vi "_Read.vi"(8 "error in (no error)":errorcluster, 11 "Lockin and Keithley Multimeter in":refnum<class "Lockin and Keithley Multimeter.lvclass">) -> (0 "error out":errorcluster, 2 "X array":T1, 3 "Lockin and Keithley Multimeter out":refnum<class "Lockin and Keithley Multimeter.lvclass">)   [LabVIEW 2017, in "Lockin and Keithley Multimeter.lvclass"]
doc: "(Protected, Dynamic, Pure Virtual/Abstract) Perform a measurement and return one or more channels of data. Outsiders should not call this method, but instead the public \"Read Data.vi\"."
uses:
  Lockin and Keithley Multimeter.lvclass
  Utility Classes/Readable/X array.ctl
  Utility Classes/Readable/X.ctl
  Lockin and Keithley Multimeter.lvclass/Lockin and Keithley Multimeter.ctl
  Lockin/sr830/SR830.lvlib
  Utility Classes/Readable/Readable.lvclass
panel:
  out "Ratio multiplier":dbl
  out "Keithley multiplier":dbl
  out "Lockin multiplier":dbl
  out "Keithley measurement":dbl format="%^.6e"
  out "R":dbl
  out "Y":dbl
  out "X":dbl
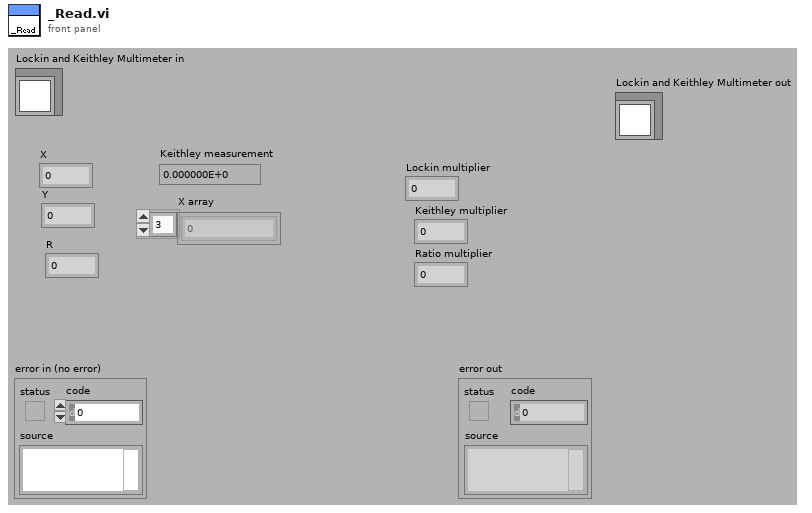
[diagram p1: front panel]
types:
  T1 = typedef "Readable.lvclass/X array.ctl" = T2[]
  T2 = typedef "Readable.lvclass/X.ctl" = dbl
  T3 = typedef "Lockin SR830.lvclass/Sensitivity.ctl" = u16
  T4 = cluster{"error":bool, "code":i32, "source":string}
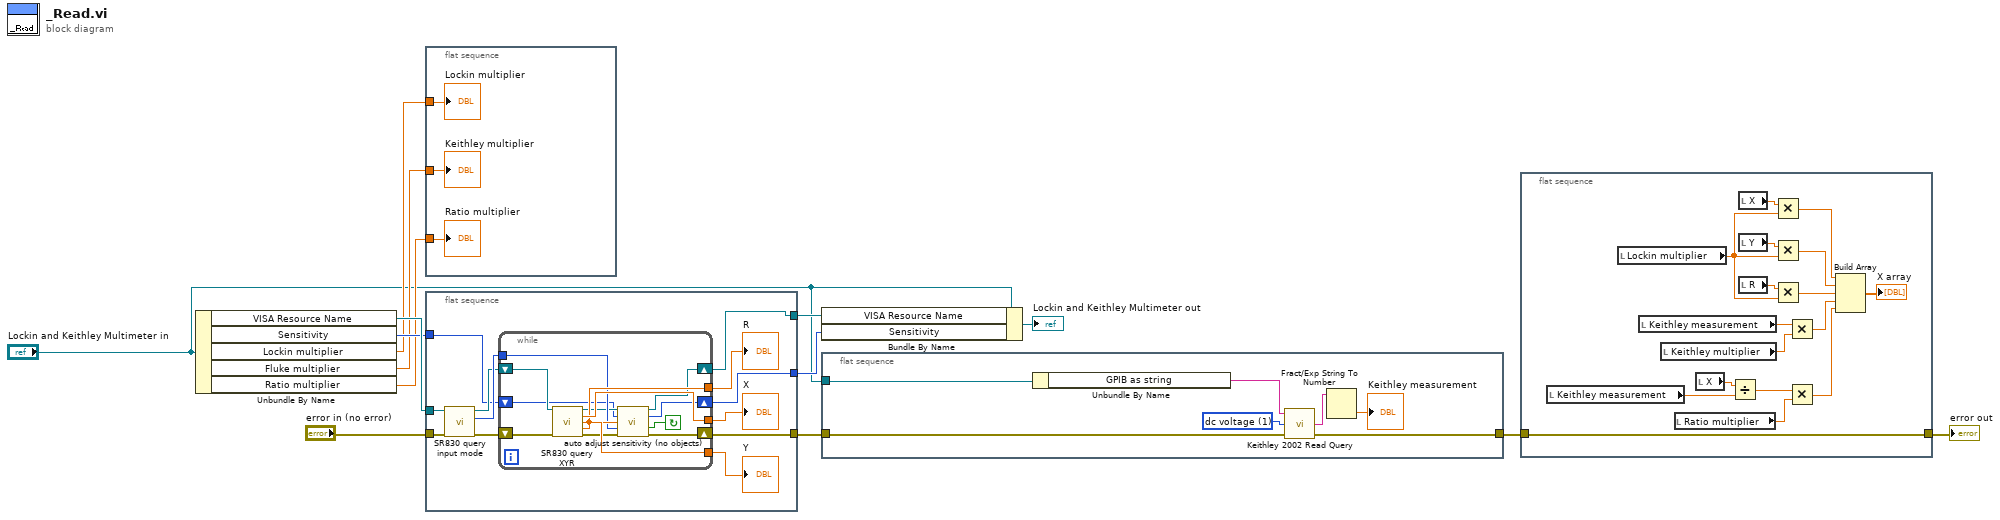
[diagram p0: block diagram]
diagram:
  n1 = Unbundle By Name("Lockin and Keithley Multimeter in") -> ("VISA Resource Name"=w13:refnum<visa-resource-name>, "Sensitivity"=w12:T3, "Lockin multiplier"=w4:dbl, "Fluke multiplier"=w5:dbl, "Ratio multiplier"=w6:dbl)
  n2 = flat-sequence {
    tunnel: w6 -> [w16]
    tunnel: w5 -> [w15]
    tunnel: w4 -> [w14]
    frame #0 {
      "Lockin multiplier" <- w14
      "Keithley multiplier" <- w15
      "Ratio multiplier" <- w16
    }
  }
  n3 = flat-sequence {
    tunnel: w13 -> [w25]
    tunnel: w12 -> [w24]
    tunnel: [w21] -> w11
    tunnel: [w20] -> w10
    tunnel: "error in (no error)" -> [w18]
    tunnel: [w17] -> w8
    frame #0 {
      n4 = call "SR830 query input mode.vi"("error in (no error)"=w18, "VISA resource name"=w25) -> ("error out"=w26:errorcluster, "input mode"=w28:enum16{"A", "A-B", "I (10^6)", "I (10^8)"}, "VISA resource name out"=w27:refnum<visa-resource-name>)  [unwired: 7 in]
      n5 = while {
        tunnel: w28 -> [w36]
        shift-right: [w29] -> w20
        shift-left: w24 -> [w30]
        shift-right: [w33] -> w17
        shift-left: w26 -> [w41]
        shift-right: [w31] -> w21
        shift-left: w27 -> [w40]
        tunnel: [w39] -> w19
        tunnel: [w38] -> w23
        tunnel: [w37] -> w22
        stop <- w34 continue-if-true
        n6 = call "SR830 query XYR.vi"("VISA resource name"=w40, "error in (no error)"=w41) -> ("VISA resource name out"=w32:refnum<visa-resource-name>, "X"=w39:dbl, "Y"=w38:dbl, "R"=w37:dbl, "error out"=w35:errorcluster)  [unwired: 9 in]
        n7 = call "auto adjust sensitivity (no objects).vi"("VISA Resource Name"=w32, "sensitivity"=w30, "R value"=w37, "Input Setting"=w36, "error in (no error)"=w35) -> ("VISA resource name out"=w31:refnum<visa-resource-name>, "sensitivity out"=w29:i8, "Repeat Measurement?"=w34:bool, "error out"=w33:errorcluster)  [unwired: 7 in]
      }
      "X" <- w19
      "Y" <- w23
      "R" <- w22
    }
  }
  n8 = Bundle By Name(cluster="Lockin and Keithley Multimeter in", "VISA Resource Name"=w11, "Sensitivity"=w10) -> (→"Lockin and Keithley Multimeter out":refnum<class "Lockin and Keithley Multimeter.lvclass">)
  n9 = flat-sequence {
    tunnel: w8 -> [w47]
    tunnel: [w48] -> w2
    tunnel: "Lockin and Keithley Multimeter in" -> [w43]
    frame #0 {
      w46 = u16 1 items=["ac voltage", "dc voltage", "2-wire resistance", "4-wire resistance", "ac current", "dc current", "frequency", "temperature"] ("function (Vdc:1)")
      n10 = Unbundle By Name(w43) -> ("GPIB as string"=w42:string)
      n11 = call "Keithley 2002 Read Query.vi"("error in"=w47, "function (Vdc:1)"=w46, "GPIB Address"=w42) -> ("error out"=w48:T4, "Reading Result"=w45:string)  [unwired: 1 in]
      n12 = Fract/Exp String To Number(string=w45) -> (number=→"Keithley measurement":dbl)  [unwired: 3 in, 1 out]
    }
  }
  n13 = flat-sequence {
    tunnel: [w49] -> w3
    tunnel: w2 -> [w49]
    frame #0 {
      n14 = local read "Keithley measurement"() -> (w56:dbl)
      n15 = local read "Lockin multiplier"() -> (w61:dbl)
      n16 = local read "Keithley measurement"() -> (w51:dbl)
      n17 = local read "Keithley multiplier"() -> (w52:dbl)
      n18 = local read "Ratio multiplier"() -> (w54:dbl)
      n19 = local read "X"() -> (w57:dbl)
      n20 = Divide(x=w57, y=w56) -> (x/y=w55:dbl)
      n21 = local read "X"() -> (w64:dbl)
      n22 = local read "Y"() -> (w63:dbl)
      n23 = local read "R"() -> (w62:dbl)
      n24 = Multiply(x=w64, y=w61) -> (x*y=w60:dbl)
      n25 = Multiply(x=w63, y=w61) -> (x*y=w59:dbl)
      n26 = Multiply(x=w62, y=w61) -> (x*y=w58:dbl)
      n27 = Multiply(x=w51, y=w52) -> (x*y=w50:dbl)
      n28 = Multiply(x=w55, y=w54) -> (x*y=w53:dbl)
      n29 = Build Array(w60, w59, w58, w50, w53) -> (→"X array":dbl[])
    }
  }
  "error out" <- w3
